vi "Register Events.vi"(0 "Display State In":T2, 9 "Container State":T3, 11 "error in (no error)":errorcluster) -> (4 "Display State Out":T2, 6 "Events":T1, 15 "error out":errorcluster)   [LabVIEW 2020, in "WebView2 XControl.lvlib" / "WebView2 Control.xctl"]
uses:
  WebView2 Control.xctl
  <vilib>/_xctls/Container State.ctl
  State.ctl
  Webview2 Lib/WebView2 Control Object/WebView2 Control.lvclass
  Webview2 Lib/WebView2 Control Object/Events.ctl
  Webview2 Lib/WebView2 Control Object/Navigation Event Data.ctl
  Webview2 Lib/WebView2 Control Object/Source Changed Event Data.ctl
  Webview2 Lib/WebView2 Control Object/Navigation Start Event Data.ctl
  Webview2 Lib/WebView2 Control Object/Read Events.vi
  <vilib>/_xctls/XControlSupport.lvlib
panel:
  # "Add Controls & Indicators that form the parameters of the method here. Hook them to the connector pane. Do not delete the controls & indicators that are already hooked to the connector pane.\n \nTo setup the parameters  for this method, right click on this item in the Project Tree & select \"Configure Method...\"."
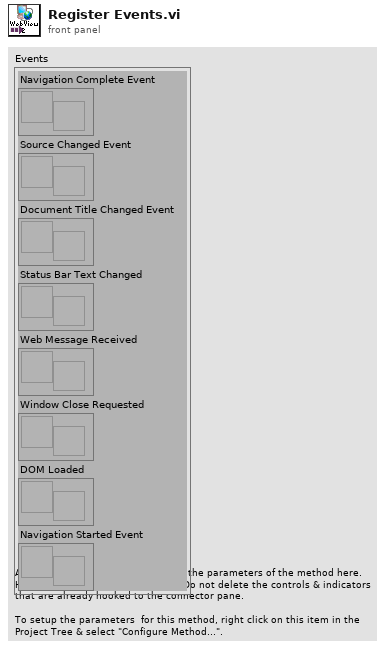
[diagram p1: front panel]
types:
  T1 = typedef "WebView2.lvlib/WebView2 Control.lvclass/Events.ctl" = cluster{"Navigation Complete Event":refnum<user-event>, "Source Changed Event":refnum<user-event>, "Document Title Changed Event":refnum<user-event>, "Status Bar Text Changed":refnum<user-event>, "Web Message Received":refnum<user-event>, "Window Close Requested":refnum<user-event>, "DOM Loaded":refnum<user-event>, "Navigation Started Event":refnum<user-event>}
  T2 = typedef "WebView2 XControl.lvlib/WebView2 Control.xctl/State.ctl" = cluster{"Control Object Ref":refnum<data-value>}
  T3 = typedef "XControlSupport.lvlib/Container State.ctl" = cluster{"Indicator?":bool, "Run Mode?":bool, " Refnum":refnum<vi>}
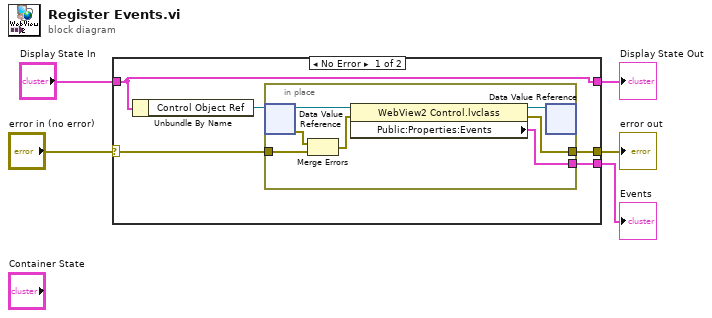
[diagram p0: block diagram]
diagram:
  n1 = case shown="No Error" "error in (no error)" {
    selector: "error in (no error)" -> [w6 w19]
    tunnel: [w10 w18] -> w2
    tunnel: "Display State In" -> [w10 w18]
    tunnel: [w8 w19] -> w4
    tunnel: [w7 _] -> w1
    frame No Error {
      n2 = Unbundle By Name(w10) -> ("Control Object Ref"=w9:refnum<data-value>)
      n3 = in-place {
        in-place-border: [w14] -> w8
        in-place-border: [w11] -> w7
        in-place-border: w6 -> [w15]
        n4 = in-place-dvr #1(w9) -> (w13:refnum<class "WebView2 Control.lvclass">, w17:errorcluster)
        n5 = Merge Errors(w17, w15) -> (w16:errorcluster)
        n6 = property class="WebView2 Control.lvclass"(reference=w13, error in=w16) -> (reference out=w12:refnum<class "WebView2 Control.lvclass">, error out=w14:errorcluster, "Public:Properties:Events"=w11:T1)
        n7 = in-place-dvr #1(w12) -> ()  [unwired: 2 out]
      }
    }
    frame Error {
    }
  }
  "Display State Out" <- w2
  "error out" <- w4
  "Events" <- w1
